vi "Status SpecimenTempCtrlSettings.vi"   [LabVIEW 2016, in "Environment Chamber.lvlib" / "Climatic Chamber.lvlib"]
uses:
  Climatic Chamber.lvlib
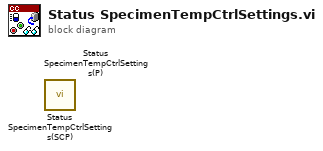
[diagram p0: block diagram]
diagram:
  n1 = call "Status SpecimenTempCtrlSettings(SCP).vi"() -> ()  [unwired: 6 in, 6 out]
  n2 = call "Status SpecimenTempCtrlSettings(P).vi"() -> ()  [unwired: 7 in, 5 out]
